vi "Read Items.vi"(8 "error in (no error)":errorcluster, 11 "Order in":refnum<class "Order.lvclass">) -> (0 "error out":errorcluster, 2 "Items":refnum<class "Beverage.lvclass">[](array[class]), 3 "Order out":refnum<class "Order.lvclass">)   [LabVIEW 2020, in "Order.lvclass"]
doc: "Simple accessor method to read the items contained in the Order."
uses:
  Order.lvclass
  Beverages/Beverage/Beverage.lvclass
  Order.lvclass/Order.ctl
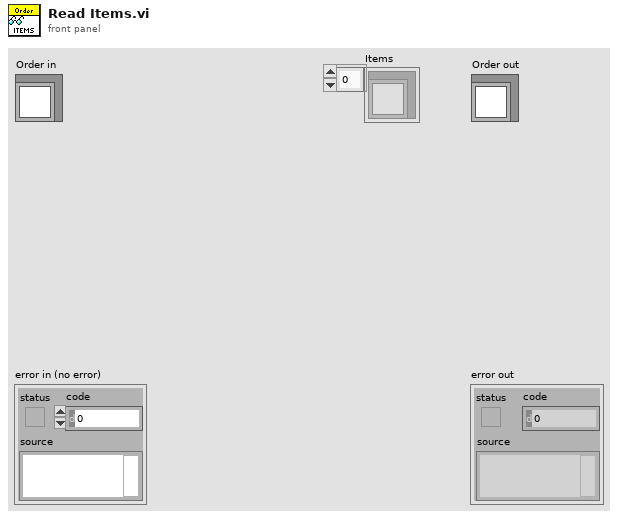
[diagram p1: front panel]
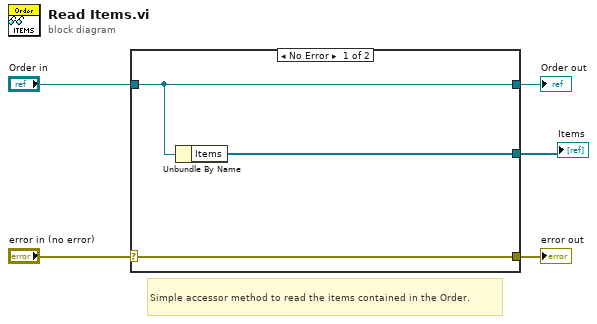
[diagram p0: block diagram]
diagram:
  # "Simple accessor method to read the items contained in the Order."
  n1 = case shown="No Error" "error in (no error)" {
    selector: "error in (no error)" -> [w8 w9]
    tunnel: [w8 w9] -> w4
    tunnel: [w7 w10] -> w2
    tunnel: "Order in" -> [w7 w10]
    tunnel: [w6 _] -> w1
    frame No Error {
      n2 = Unbundle By Name(w7) -> ("Items"=w6:refnum<class "Beverage.lvclass">[])
    }
    frame Error {
    }
  }
  "error out" <- w4
  "Order out" <- w2
  "Items" <- w1
